vi "Update Configuration.vi"(8 "error in (no error)":errorcluster, 11 "CIFPlugin in":refnum<class "Template_Plugin.lvclass">) -> (0 "error out":errorcluster, 3 "CIFPlugin out":refnum<class "Template_Plugin.lvclass">)   [LabVIEW 2021, in "Template_Plugin.lvclass"]
uses:
  Template_Plugin.lvclass
  C:/Program Files/National Instruments/LabVIEW 2021/vi.lib/CIF Foundation/CIF Core/CIFCore/Class/CIFCorePlugin.lvclass
  <vilib>/CIF Foundation/CIF Core/CIFCore/Class/CIFCorePlugin.lvclass/CIFCorePlugin.ctl
  Template_Plugin.lvclass/Template_Plugin.ctl
  <vilib>/CIF Foundation/CIF Core/CIFCore/Class/CIFCorePlugin.lvclass
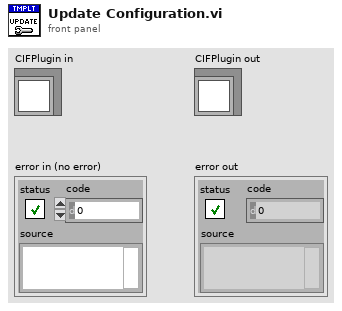
[diagram p1: front panel]
types:
  T1 = typedef "Template_Common.lvlib/Configuration.ctl" = cluster{"Common":T2, "Step":u64}
  T2 = typedef "CIFCoreCommon.lvlib/Common Plugin Configuration.ctl" = cluster{"Period (s)":dbl, "Offset (us)":i32, "ClockID":u8, "Priority":i32, "Processor":i32}
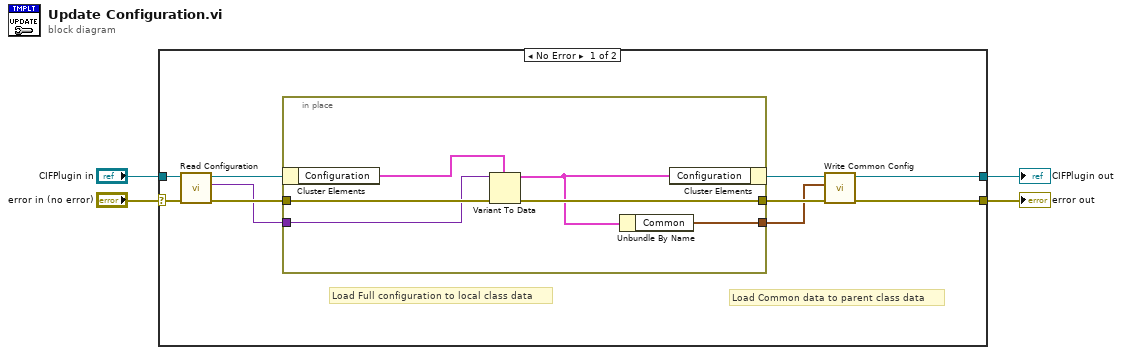
[diagram p0: block diagram]
diagram:
  n1 = case shown="No Error" "error in (no error)" {
    selector: "error in (no error)" -> [w8 w21]
    tunnel: "CIFPlugin in" -> [w9 w22]
    tunnel: [w10 w22] -> w1
    tunnel: [w11 w21] -> w3
    frame No Error {
      # "Load Common data to parent class data"
      # "Load Full configuration to local class data"
      n2 = call <vilib>:"Read Configuration.vi"("error in"=w8, "CIFCorePlugin in"=w9) -> ("error out"=w7:errorcluster, "Configuration Data"=w6:variant, "CIFCorePlugin out"=w5:refnum<class "Template_Plugin.lvclass">)  [unwired: 7 in]
      n3 = in-place {
        in-place-border: [w20] -> w14
        in-place-border: w7 -> [w19]
        in-place-border: w6 -> [w18]
        in-place-border: [w16] -> w13
        n4 = in-place-cluster #1(w5) -> ("Configuration"=w17:T1)
        n5 = Variant To Data(error in=w19, type=w17, Variant=w18) -> (data=w15:T1, error out=w20:errorcluster)
        n6 = Unbundle By Name(w15) -> ("Common"=w16:T2)
        n7 = in-place-cluster #1("Configuration"=w15) -> (w12:refnum<class "Template_Plugin.lvclass">)
      }
      n8 = call <vilib>:"Write Common Config.vi"("error in (no error)"=w14, "Common"=w13, "CIFTemplateNode in"=w12) -> ("error out"=w11:errorcluster, "CIFTemplateNode out"=w10:refnum<class "Template_Plugin.lvclass">)  [unwired: 7 in]
    }
    frame Error {
    }
  }
  "error out" <- w3
  "CIFPlugin out" <- w1
